vi "IMU_Process_Data.vi"(8 "error in (no error)":errorcluster caption="Fehler (Eingang, kein Fehler)", 10 "Received Raw Data Byte-Array U8":u8[](array[numeric]), 11 "MultiWii Data Cluster 2":refnum<vi>) -> (0 "error out":errorcluster caption="Fehler (Ausgang)")   [LabVIEW 2017]
uses:
  IMU_Data_Cluster.ctl
  <vilib>/Analysis/baseanly.llb/Mean (DBL).vi
  <vilib>/Analysis/NI_AALBase.lvlib
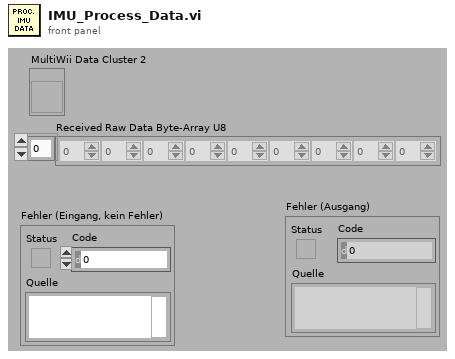
[diagram p1: front panel]
types:
  T1 = typedef "IMU_Data_Cluster.ctl" = cluster{"Firmware Revision":string, "Multitype Name":string, "Cycle Time":u16, "I²C Error Count":u16, "ACC present":bool, "Baro present":bool, "Mag Present":bool, "GPS present":bool, "Sonar present":bool, "Acc X axis (Roll)":dbl, "Acc Y axis (Pitch)":dbl, "Acc Z axis (Yaw)":dbl, "Gyro X axis (Roll)":dbl, "Gyro Y axis (Pitch)":dbl, "Gyro Z axis (Yaw)":dbl, "Mag X axis (Roll)":dbl, "Mag Y axis (Pitch)":dbl, "Mag Z axis (Yaw)":dbl, "X angle (Roll)":dbl, "Y angle (Pitch)":dbl, "Heading [°]":dbl, "Altitude [m]":dbl, "Vario":dbl, "GPS_Fix":u8, "GPS_NumSat":u8, "GPS_coord[LAT]":dbl, "GPS_coord[LON]":dbl, "GPS_Altitude":dbl, "GPS_Speed over Ground":dbl, "GPS_Ground Course":dbl, "Baro P [mbara]":dbl, "Baro T [°C]":dbl, "Altitude abs [m]":dbl}
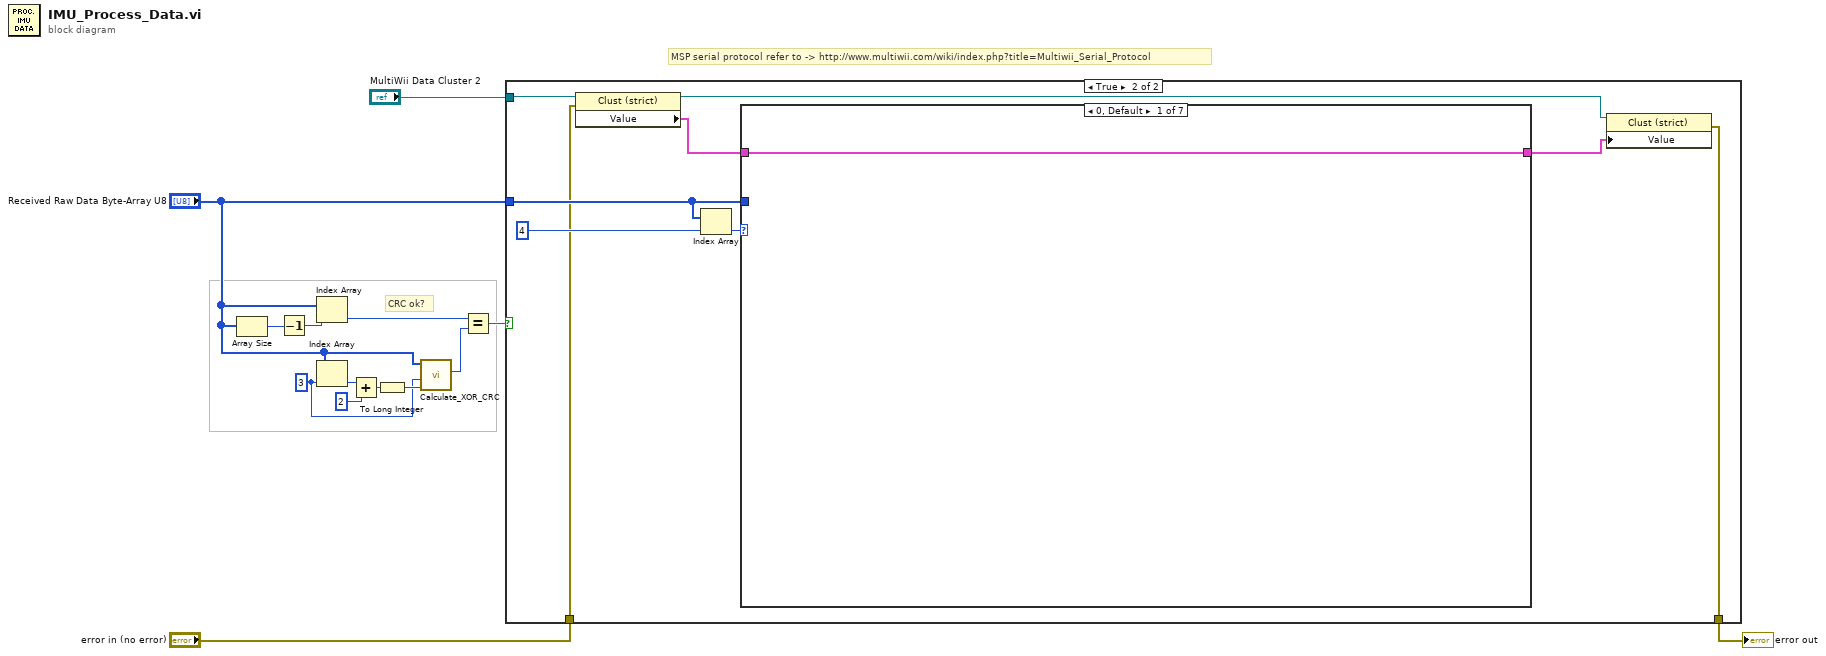
[diagram p0: block diagram]
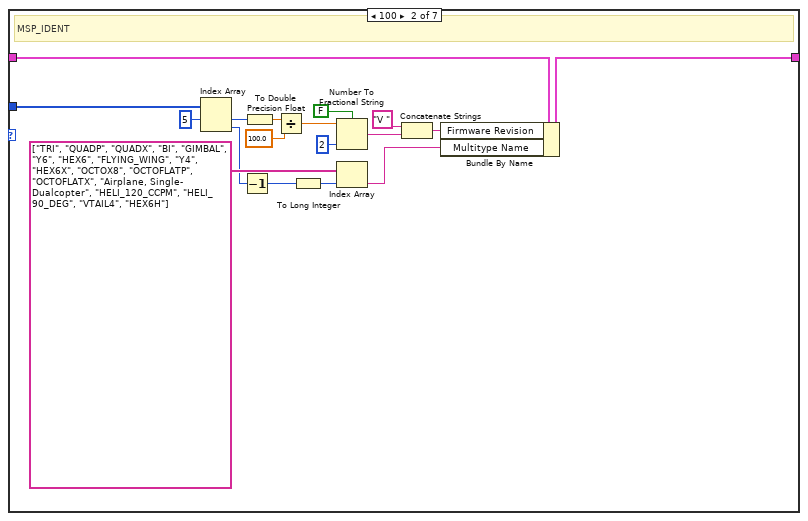
[diagram p3: hidden frame]
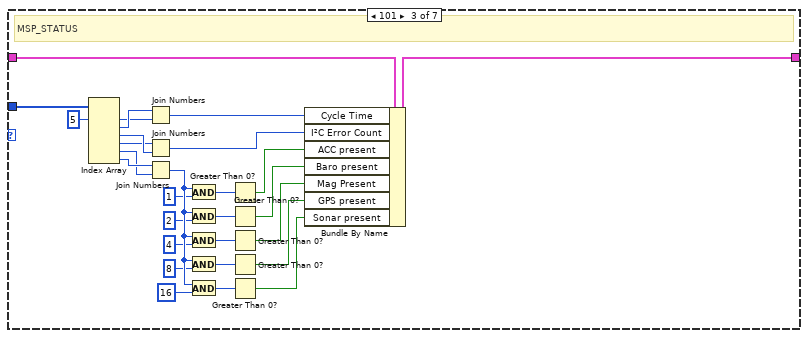
[diagram p4: hidden frame]
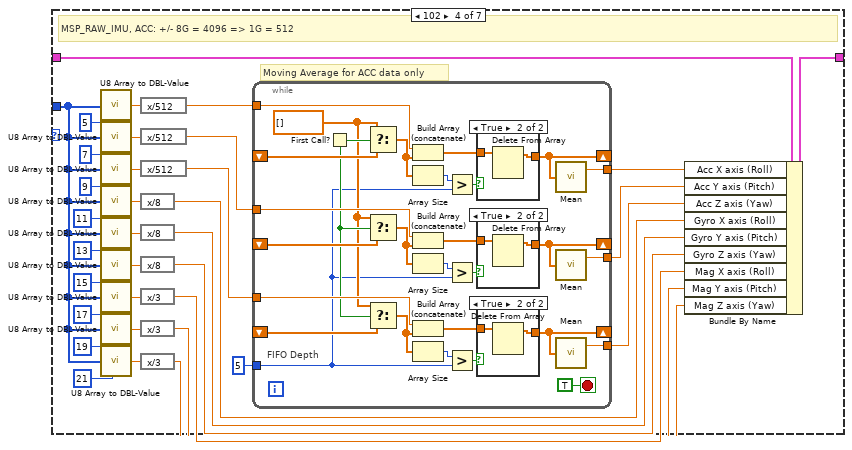
[diagram p5: hidden frame]
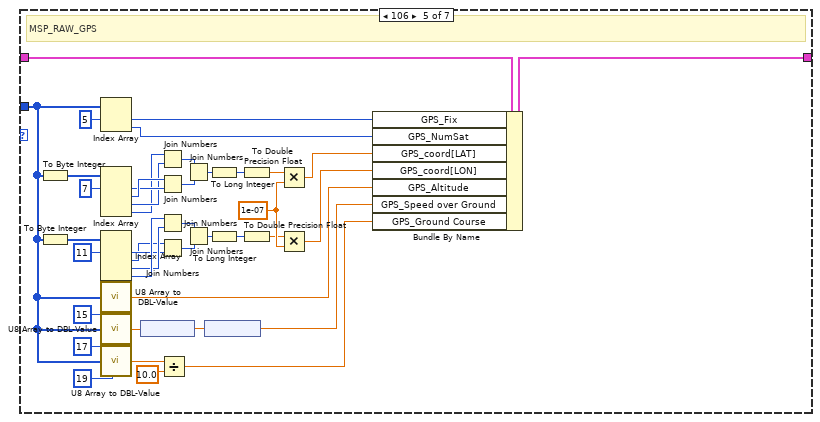
[diagram p9: hidden frame]
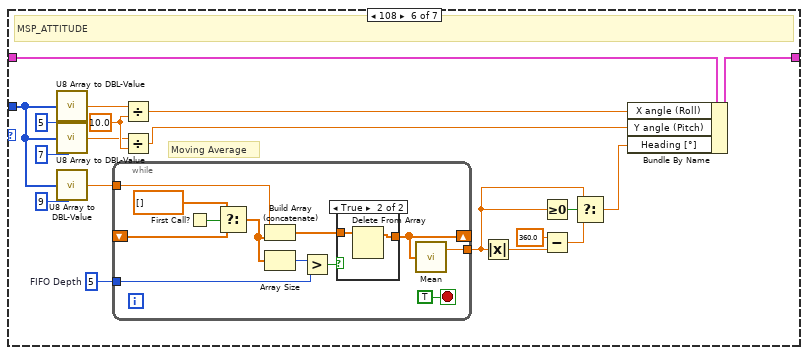
[diagram p10: hidden frame]
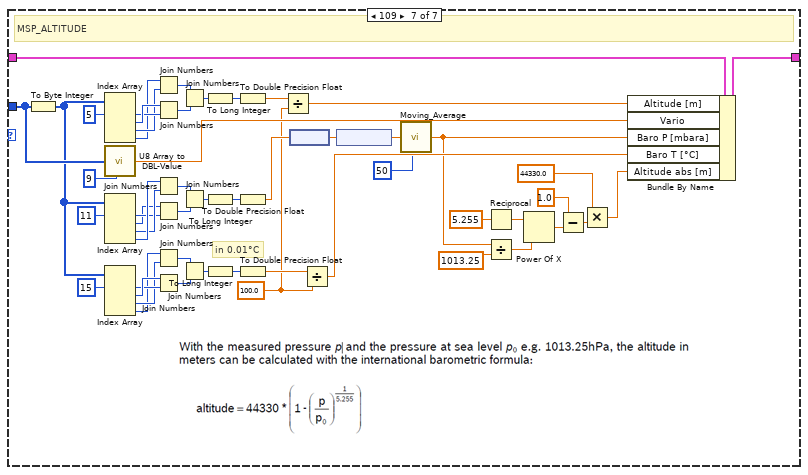
[diagram p12: hidden frame]
diagram:
  w8 = 3 ("Index")
  # "MSP serial protocol refer to -> http://www.multiwii.com/wiki/index.php?title=Multiwii_Serial_Protocol"
  # "CRC ok?"
  n1 = Array Size(array="Received Raw Data Byte-Array U8") -> (size(s)=w14:i32)
  n2 = Decrement(x=w14) -> (x-1=w13:i32)
  n3 = Index Array(array="Received Raw Data Byte-Array U8", index=w13) -> (element=w7:u8)
  n4 = Index Array(array="Received Raw Data Byte-Array U8", index=w8) -> (element=w12:u8)
  n5 = Add(x=w12, y=u8 2) -> (x+y=w10:u8)
  n6 = To Long Integer(number=w10) -> (32bit integer=w9:i32)
  n7 = call "Calculate_XOR_CRC.vi"("No. of Bytes for Calculation"=w9, "Start Position (Byte)"=w8, "U8 Byte Array"="Received Raw Data Byte-Array U8") -> ("CRC"=w6:u8)  [unwired: 8 in]
  n8 = Equal?(x=w7, y=w6) -> (x = y?=w4:bool)
  n9 = case shown="True" w4 {
    tunnel: "Received Raw Data Byte-Array U8" -> [_ w24]
    tunnel: "MultiWii Data Cluster 2" -> [_ w21]
    tunnel: "error in (no error)" -> [w15 w17]
    tunnel: [w15 w16] -> w1
    frame False {
    }
    frame True {
      n10 = property class="Clust (strict)"(reference=w21, error in=w17) -> (reference out=w19:refnum<vi>, "Value"=w20:T1)  [unwired: 1 out]
      n11 = Index Array(array=w24, index=4 ("Index")) -> (element=w22:u8)
      n12 = case shown="0, Default" w22 {
        tunnel: w24 -> [_ w30 w57 w105 w155 w197 w258]
        tunnel: w20 -> [w25 w27 w56 w79 w182 w201 w261]
        tunnel: [w25 w26 w55 w85 w181 w200 w260] -> w18
        frame 0, Default {
        }
        frame 100 {
          # "MSP_IDENT"
          n13 = Index Array(array=w30, index #1=5 ("Index")) -> (element #1=w39:u8, element #2=w41:u8)  [unwired: 1 in]
          n14 = Decrement(x=w41) -> (x-1=w33:u8)
          n15 = To Double Precision Float(number=w39) -> (double precision float=w38:dbl)
          n16 = Divide(x=w38, y=100.0) -> (x/y=w36:dbl)
          n17 = To Long Integer(number=w33) -> (32bit integer=w40:i32)
          n18 = Number To Fractional String(use system decimal point (T)=FALSE ("Systemdezimalzeichen verwenden (T)"), number=w36, precision (6)=i16 2 ("Genauigkeit (6)")) -> (F-format string=w32:string)  [unwired: 1 in]
          n19 = Index Array(array=string[] ["TRI", "QUADP", "QUADX", "BI", "GIMBAL", "Y6", "HEX6", "FLYING_WING", "Y4", "HEX6X", "OCTOX8", "OCTOFLATP", "OCTOFLATX", "Airplane, Single- Dualcopter", "HELI_120_CCPM", "HELI_90_DEG", "VTAIL4", "HEX6H"], index=w40) -> (element=w28:string)
          n20 = Concatenate Strings("V " ("String"), w32) -> (w29:string)
          n21 = Bundle By Name(cluster=w27, "Firmware Revision"=w29, "Multitype Name"=w28) -> (w26:T1)
        }
        frame 101 {
          # "MSP_STATUS"
          n22 = Index Array(array=w57, index #1=5 ("Index")) -> (element #1=w58:u8, element #2=w59:u8, element #3=w47:u8, element #4=w46:u8, element #5=w44:u8, element #6=w45:u8)  [unwired: 5 in]
          n23 = Join Numbers(hi=w59, lo=w58) -> ((hi.lo)=w54:u16)
          n24 = Join Numbers(hi=w46, lo=w47) -> ((hi.lo)=w53:u16)
          n25 = Join Numbers(hi=w45, lo=w44) -> ((hi.lo)=w71:u16)
          n26 = And(x=w71, y=u16 1) -> (x .and. y?=w62:u16)
          n27 = And(x=w71, y=u16 2) -> (x .and. y?=w63:u16)
          n28 = And(x=w71, y=u16 4) -> (x .and. y?=w66:u16)
          n29 = And(x=w71, y=u16 8) -> (x .and. y?=w67:u16)
          n30 = And(x=w71, y=u16 16) -> (x .and. y?=w70:u16)
          n31 = Greater Than 0?(x=w62) -> (x > 0?=w52:bool)
          n32 = Greater Than 0?(x=w63) -> (x > 0?=w51:bool)
          n33 = Greater Than 0?(x=w66) -> (x > 0?=w50:bool)
          n34 = Greater Than 0?(x=w67) -> (x > 0?=w49:bool)
          n35 = Greater Than 0?(x=w70) -> (x > 0?=w48:bool)
          n36 = Bundle By Name(cluster=w56, "Cycle Time"=w54, "I²C Error Count"=w53, "ACC present"=w52, "Baro present"=w51, "Mag Present"=w50, "GPS present"=w49, "Sonar present"=w48) -> (w55:T1)
        }
        frame 102 {
          # "Moving Average for ACC data only"
          # "MSP_RAW_IMU, ACC: +/- 8G = 4096 => 1G = 512"
          n37 = call "U8 Array to DBL-Value.vi"("IMU Data Array U8"=w105, "pos.=lowbyte, pos.+1=highbyte"=5 ("Index")) -> ("Data Value (DBL)"=w95:dbl)  [unwired: 5 in]
          n38 = call "U8 Array to DBL-Value.vi"("IMU Data Array U8"=w105, "pos.=lowbyte, pos.+1=highbyte"=7 ("Index")) -> ("Data Value (DBL)"=w94:dbl)  [unwired: 5 in]
          n39 = call "U8 Array to DBL-Value.vi"("IMU Data Array U8"=w105, "pos.=lowbyte, pos.+1=highbyte"=9 ("Index")) -> ("Data Value (DBL)"=w93:dbl)  [unwired: 5 in]
          n40 = call "U8 Array to DBL-Value.vi"("IMU Data Array U8"=w105, "pos.=lowbyte, pos.+1=highbyte"=11 ("Index")) -> ("Data Value (DBL)"=w90:dbl)  [unwired: 5 in]
          n41 = call "U8 Array to DBL-Value.vi"("IMU Data Array U8"=w105, "pos.=lowbyte, pos.+1=highbyte"=13 ("Index")) -> ("Data Value (DBL)"=w92:dbl)  [unwired: 5 in]
          n42 = call "U8 Array to DBL-Value.vi"("IMU Data Array U8"=w105, "pos.=lowbyte, pos.+1=highbyte"=15 ("Index")) -> ("Data Value (DBL)"=w91:dbl)  [unwired: 5 in]
          n43 = call "U8 Array to DBL-Value.vi"("IMU Data Array U8"=w105, "pos.=lowbyte, pos.+1=highbyte"=17 ("Index")) -> ("Data Value (DBL)"=w89:dbl)  [unwired: 5 in]
          n44 = call "U8 Array to DBL-Value.vi"("IMU Data Array U8"=w105, "pos.=lowbyte, pos.+1=highbyte"=19 ("Index")) -> ("Data Value (DBL)"=w88:dbl)  [unwired: 5 in]
          n45 = call "U8 Array to DBL-Value.vi"("IMU Data Array U8"=w105, "pos.=lowbyte, pos.+1=highbyte"=21 ("Index")) -> ("Data Value (DBL)"=w87:dbl)  [unwired: 5 in]
          n46 = expression code="x/512"(w95) -> (w86:dbl)
          n47 = expression code="x/512"(w94) -> (w83:dbl)
          n48 = expression code="x/512"(w93) -> (w81:dbl)
          n49 = expression code="x/8"(w90) -> (w77:dbl)
          n50 = expression code="x/8"(w92) -> (w76:dbl)
          n51 = expression code="x/8"(w91) -> (w75:dbl)
          n52 = expression code="x/3"(w89) -> (w74:dbl)
          n53 = expression code="x/3"(w88) -> (w73:dbl)
          n54 = expression code="x/3"(w87) -> (w72:dbl)
          n55 = while {
            shift-right: [w133] -> _
            shift-left: _ -> [w129]
            tunnel: [w126] -> w84
            tunnel: w86 -> [w125]
            shift-right: [w117] -> _
            shift-left: _ -> [w121]
            tunnel: [w123] -> w82
            tunnel: w83 -> [w124]
            shift-right: [w116] -> _
            shift-left: _ -> [w112]
            tunnel: [w110] -> w80
            tunnel: w81 -> [w109]
            tunnel: 5 ("FIFO-Size") -> [w106]
            stop <- TRUE stop-if-true
            w107 = dbl[] []
            # "FIFO Depth"
            n56 = First Call?() -> (First Call?: T/F=w108:bool)
            n57 = Select(t=w107, s=w108, f=w129) -> (s? t:f=w128:dbl[])
            n58 = Select(t=w107, s=w108, f=w121) -> (s? t:f=w122:dbl[])
            n59 = Select(t=w107, s=w108, f=w112) -> (s? t:f=w111:dbl[])
            n60 = Build Array (concatenate)(w125, w128) -> (w130:dbl[])
            n61 = Array Size(array=w128) -> (size(s)=w132:i32)
            n62 = Build Array (concatenate)(w124, w122) -> (w120:dbl[])
            n63 = Array Size(array=w122) -> (size(s)=w118:i32)
            n64 = Build Array (concatenate)(w109, w111) -> (w113:dbl[])
            n65 = Array Size(array=w111) -> (size(s)=w115:i32)
            n66 = Greater?(x=w132, y=w106) -> (0:w131:bool)
            n67 = Greater?(x=w118, y=w106) -> (0:w119:bool)
            n68 = Greater?(x=w115, y=w106) -> (0:w114:bool)
            n69 = case shown="True" w131 {
              tunnel: [w140 w141] -> w133
              tunnel: w130 -> [w140 w142]
              frame False {
              }
              frame True {
                n70 = Delete From Array(array=w142) -> (array with subset deleted=w141:dbl[])  [unwired: 2 in, 1 out]
              }
            }
            n71 = case shown="True" w119 {
              tunnel: [w137 w138] -> w117
              tunnel: w120 -> [w137 w139]
              frame False {
              }
              frame True {
                n72 = Delete From Array(array=w139) -> (array with subset deleted=w138:dbl[])  [unwired: 2 in, 1 out]
              }
            }
            n73 = case shown="True" w114 {
              tunnel: [w134 w135] -> w116
              tunnel: w113 -> [w134 w136]
              frame False {
              }
              frame True {
                n74 = Delete From Array(array=w136) -> (array with subset deleted=w135:dbl[])  [unwired: 2 in, 1 out]
              }
            }
            n75 = call-poly <vilib>:"Mean.vi"("X"=w133) -> ("mean"=w126:dbl)  [unwired: 1 out]
            n76 = call-poly <vilib>:"Mean.vi"("X"=w117) -> ("mean"=w123:dbl)  [unwired: 1 out]
            n77 = call-poly <vilib>:"Mean.vi"("X"=w116) -> ("mean"=w110:dbl)  [unwired: 1 out]
          }
          n78 = Bundle By Name(cluster=w79, "Acc X axis (Roll)"=w84, "Acc Y axis (Pitch)"=w82, "Acc Z axis (Yaw)"=w80, "Gyro X axis (Roll)"=w77, "Gyro Y axis (Pitch)"=w76, "Gyro Z axis (Yaw)"=w75, "Mag X axis (Roll)"=w74, "Mag Y axis (Pitch)"=w73, "Mag Z axis (Yaw)"=w72) -> (w85:T1)
        }
        frame 106 {
          w145 = 1e-07
          # "MSP_RAW_GPS"
          n79 = To Byte Integer(number=w155) -> (8bit integer=w159:i8[])
          n80 = To Byte Integer(number=w155) -> (8bit integer=w176:i8[])
          n81 = Index Array(array=w155, index #1=5 ("Index")) -> (element #1=w180:u8, element #2=w179:u8)  [unwired: 1 in]
          n82 = Index Array(array=w159, index #1=7 ("Index")) -> (element #1=w165:i8, element #2=w166:i8, element #3=w164:i8, element #4=w163:i8)  [unwired: 3 in]
          n83 = Index Array(array=w176, index #1=11 ("Index")) -> (element #1=w170:i8, element #2=w169:i8, element #3=w171:i8, element #4=w172:i8)  [unwired: 3 in]
          n84 = call "U8 Array to DBL-Value.vi"("IMU Data Array U8"=w155, "pos.=lowbyte, pos.+1=highbyte"=15) -> ("Data Value (DBL)"=w154:dbl)  [unwired: 5 in]
          n85 = call "U8 Array to DBL-Value.vi"("IMU Data Array U8"=w155, "pos.=lowbyte, pos.+1=highbyte"=17) -> ("Data Value (DBL)"=w152:dbl)  [unwired: 5 in]
          n86 = call "U8 Array to DBL-Value.vi"("IMU Data Array U8"=w155, "pos.=lowbyte, pos.+1=highbyte"=19) -> ("Data Value (DBL)"=w150:dbl)  [unwired: 5 in]
          n87 = node(w152) -> (w153:dbl[unit])
          n88 = Join Numbers(hi=w163, lo=w164) -> ((hi.lo)=w161:u16)
          n89 = Join Numbers(hi=w166, lo=w165) -> ((hi.lo)=w162:u16)
          n90 = Join Numbers(hi=w172, lo=w171) -> ((hi.lo)=w174:u16)
          n91 = Join Numbers(hi=w169, lo=w170) -> ((hi.lo)=w173:u16)
          n92 = Divide(x=w150, y=10.0) -> (x/y=w148:dbl)
          n93 = Join Numbers(hi=w161, lo=w162) -> ((hi.lo)=w160:u32)
          n94 = Join Numbers(hi=w174, lo=w173) -> ((hi.lo)=w175:u32)
          n95 = node(w153) -> (w151:dbl)
          n96 = To Long Integer(number=w160) -> (32bit integer=w158:i32)
          n97 = To Long Integer(number=w175) -> (32bit integer=w177:i32)
          n98 = To Double Precision Float(number=w158) -> (double precision float=w147:dbl)
          n99 = To Double Precision Float(number=w177) -> (double precision float=w144:dbl)
          n100 = Multiply(x=w147, y=w145) -> (x*y=w146:dbl)
          n101 = Multiply(x=w144, y=w145) -> (x*y=w143:dbl)
          n102 = Bundle By Name(cluster=w182, "GPS_Fix"=w180, "GPS_NumSat"=w179, "GPS_coord[LAT]"=w146, "GPS_coord[LON]"=w143, "GPS_Altitude"=w154, "GPS_Speed over Ground"=w151, "GPS_Ground Course"=w148) -> (w181:T1)
        }
        frame 108 {
          w186 = 5  # FIFO Depth
          w202 = 10.0 ("y")
          # "Moving Average"
          # "MSP_ATTITUDE"
          n103 = call "U8 Array to DBL-Value.vi"("IMU Data Array U8"=w197, "pos.=lowbyte, pos.+1=highbyte"=5 ("Index")) -> ("Data Value (DBL)"=w193:dbl)  [unwired: 5 in]
          n104 = call "U8 Array to DBL-Value.vi"("IMU Data Array U8"=w197, "pos.=lowbyte, pos.+1=highbyte"=7 ("Index")) -> ("Data Value (DBL)"=w192:dbl)  [unwired: 5 in]
          n105 = call "U8 Array to DBL-Value.vi"("IMU Data Array U8"=w197, "pos.=lowbyte, pos.+1=highbyte"=9 ("Index")) -> ("Data Value (DBL)"=w185:dbl)  [unwired: 5 in]
          n106 = while {
            shift-right: [w214] -> _
            shift-left: _ -> [w208]
            tunnel: [w205] -> w184
            tunnel: w185 -> [w204]
            tunnel: w186 -> [w203]
            stop <- TRUE stop-if-true
            n107 = First Call?() -> (First Call?: T/F=w210:bool)
            n108 = Select(t=dbl[] [], s=w210, f=w208) -> (s? t:f=w207:dbl[])
            n109 = Build Array (concatenate)(w204, w207) -> (w211:dbl[])
            n110 = Array Size(array=w207) -> (size(s)=w213:i32)
            n111 = Greater?(x=w213, y=w203) -> (0:w212:bool)
            n112 = case shown="True" w212 {
              tunnel: [w215 w216] -> w214
              tunnel: w211 -> [w215 w217]
              frame False {
              }
              frame True {
                n113 = Delete From Array(array=w217) -> (array with subset deleted=w216:dbl[])  [unwired: 2 in, 1 out]
              }
            }
            n114 = call-poly <vilib>:"Mean.vi"("X"=w214) -> ("mean"=w205:dbl)  [unwired: 1 out]
          }
          n115 = Divide(x=w193, y=w202) -> (x/y=w199:dbl)
          n116 = Divide(x=w192, y=w202) -> (x/y=w198:dbl)
          n117 = Absolute Value(x=w184) -> (abs(x)=w191:dbl)
          n118 = Greater Or Equal To 0?(x=w184) -> (x >= 0?=w188:bool)
          n119 = Subtract(x=360.0, y=w191) -> (x-y=w189:dbl)
          n120 = Select(t=w184, s=w188, f=w189) -> (s? t:f=w187:dbl)
          n121 = Bundle By Name(cluster=w201, "X angle (Roll)"=w199, "Y angle (Pitch)"=w198, "Heading [°]"=w187) -> (w200:T1)
        }
        frame 109 {
          w218 = 100.0 ("y")
          # "in 0.01°C"
          # "MSP_ALTITUDE"
          n122 = To Byte Integer(number=w258) -> (8bit integer=w241:i8[])
          n123 = Index Array(array=w241, index #1=5 ("Index")) -> (element #1=w267:i8, element #2=w268:i8, element #3=w266:i8, element #4=w265:i8)  [unwired: 3 in]
          n124 = call "U8 Array to DBL-Value.vi"("IMU Data Array U8"=w258, "pos.=lowbyte, pos.+1=highbyte"=9) -> ("Data Value (DBL)"=w256:dbl)  [unwired: 5 in]
          n125 = Index Array(array=w241, index #1=11 ("Index")) -> (element #1=w251:i8, element #2=w250:i8, element #3=w252:i8, element #4=w253:i8)  [unwired: 3 in]
          n126 = Index Array(array=w241, index #1=15 ("Index")) -> (element #1=w246:i8, element #2=w247:i8, element #3=w245:i8, element #4=w244:i8)  [unwired: 3 in]
          n127 = Join Numbers(hi=w265, lo=w266) -> ((hi.lo)=w263:u16)
          n128 = Join Numbers(hi=w268, lo=w267) -> ((hi.lo)=w264:u16)
          n129 = Join Numbers(hi=w253, lo=w252) -> ((hi.lo)=w255:u16)
          n130 = Join Numbers(hi=w250, lo=w251) -> ((hi.lo)=w254:u16)
          n131 = Join Numbers(hi=w244, lo=w245) -> ((hi.lo)=w242:u16)
          n132 = Join Numbers(hi=w247, lo=w246) -> ((hi.lo)=w243:u16)
          n133 = Join Numbers(hi=w263, lo=w264) -> ((hi.lo)=w262:u32)
          n134 = Join Numbers(hi=w255, lo=w254) -> ((hi.lo)=w240:u32)
          n135 = Join Numbers(hi=w242, lo=w243) -> ((hi.lo)=w238:u32)
          n136 = To Long Integer(number=w262) -> (32bit integer=w259:i32)
          n137 = To Long Integer(number=w240) -> (32bit integer=w239:i32)
          n138 = To Long Integer(number=w238) -> (32bit integer=w237:i32)
          n139 = To Double Precision Float(number=w259) -> (double precision float=w220:dbl)
          n140 = To Double Precision Float(number=w239) -> (double precision float=w224:dbl)
          n141 = To Double Precision Float(number=w237) -> (double precision float=w227:dbl)
          n142 = Divide(x=w220, y=w218) -> (x/y=w219:dbl)
          n143 = node(w224) -> (w225:dbl[unit])
          n144 = Divide(x=w227, y=w218) -> (x/y=w226:dbl)
          n145 = node(w225) -> (w223:dbl)
          n146 = call "Moving_Average.vi"("Sensor Value"=w223, "FIFO-Size"=50) -> ("Moving Average"=w222:dbl)  [unwired: 5 in]
          n147 = Reciprocal(x=5.255) -> (1/x=w229:dbl)
          n148 = Divide(x=w222, y=1013.25) -> (x/y=w234:dbl)
          n149 = Power Of X(1:w234, 2:w229) -> (0:w233:dbl)
          n150 = Subtract(x=1.0, y=w233) -> (x-y=w230:dbl)
          n151 = Multiply(x=44330.0, y=w230) -> (x*y=w228:dbl)
          n152 = Bundle By Name(cluster=w261, "Altitude [m]"=w219, "Vario"=w256, "Baro P [mbara]"=w222, "Baro T [°C]"=w226, "Altitude abs [m]"=w228) -> (w260:T1)
        }
      }
      n153 = property class="Clust (strict)"(reference=w19, "Value"=w18) -> (error out=w16:errorcluster)  [unwired: 1 in, 1 out]
    }
  }
  "error out" <- w1
